vi "Device Params 2 Config XML File.vi"(8 "error IN":errorcluster, 9 "Device Settings":T1, 10 "Device Connections":T2, 11 "Configuration in":refnum<class "Configuration.lvclass">) -> (0 "error OUT":errorcluster, 3 "Configuration out":refnum<class "Configuration.lvclass">)   [LabVIEW 2011]
uses:
  Controls/Device Connections.ctl
  Controls/Device Settings.ctl
  Modules/File/Configuration/Configuration.lvclass
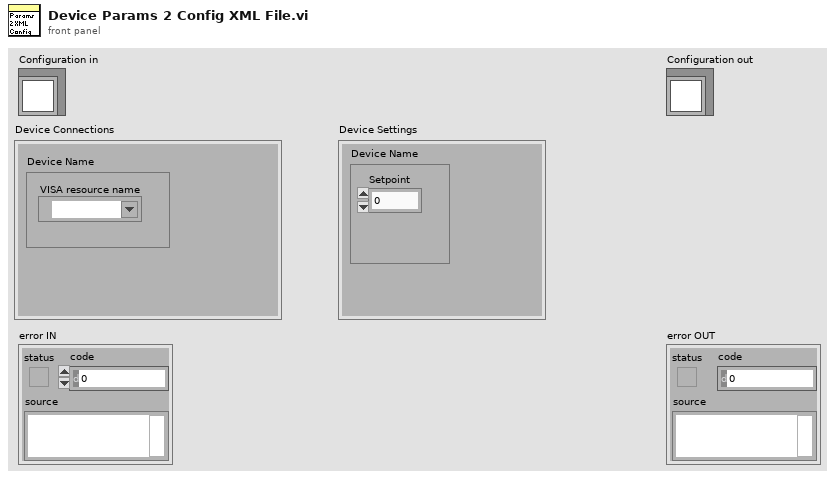
[diagram p1: front panel]
types:
  T1 = typedef "Device Settings.ctl" = cluster{"Device Name":cluster{"Setpoint":dbl}}
  T2 = typedef "Device Connections.ctl" = cluster{"Device Name":cluster{"VISA resource name":refnum<visa-resource-name>}}
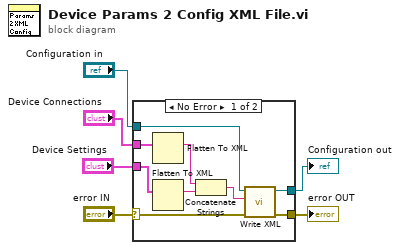
[diagram p0: block diagram]
diagram:
  n1 = case shown="No Error" "error IN" {
    selector: "error IN" -> [w15 w16]
    tunnel: [w7 w17] -> w3
    tunnel: "Configuration in" -> [w14 w17]
    tunnel: [w8 w16] -> w1
    tunnel: "Device Connections" -> [w13 _]
    tunnel: "Device Settings" -> [w12 _]
    frame No Error {
      n2 = Flatten To XML(anything=w13) -> (xml string=w11:string)
      n3 = Flatten To XML(anything=w12) -> (xml string=w10:string)
      n4 = Concatenate Strings(w11, w10) -> (w9:string)
      n5 = call-dynamic "Write XML.vi"("error in (no error)"=w15, "String"=w9, "Configuration in"=w14) -> ("error out"=w8:errorcluster, "Configuration out"=w7:refnum<class "Configuration.lvclass">)  [unwired: 7 in]
    }
    frame Error {
    }
  }
  "Configuration out" <- w3
  "error OUT" <- w1
